vi "User_Controls.vi"() -> ()   [LabVIEW 2024]
uses:
  <vilib>/MakerHub/LINX/Public/Peripherals/Analog/Analog Read 1 Chan.vi
  <vilib>/MakerHub/LINX/Public/Peripherals/Digital/Digital Write 1 Chan.vi
  <vilib>/MakerHub/LINX/Public/Peripherals/Digital/Digital Read 1 Chan.vi
  <vilib>/MakerHub/LINX/Public/Peripherals/PWM/PWM Set Duty Cycle 1 Chan.vi
  <vilib>/MakerHub/LINX/Public/Peripherals/Digital/Digital Write N Chans.vi
  <vilib>/MakerHub/LINX/Public/Peripherals/Analog/Analog Read N Chans.vi
  <vilib>/MakerHub/LINX/Public/Peripherals/Digital/Digital Read N Chans.vi
  <vilib>/MakerHub/LINX/Private/Local IO/LinxDigitalWrite.vi
  <vilib>/MakerHub/LINX/Public/Utilities/Check Channel.vi
  <vilib>/MakerHub/LINX/Private/Local IO/LinxAnalogRead.vi
  <vilib>/MakerHub/LINX/Private/Local IO/LinxDigitalRead.vi
  <vilib>/MakerHub/LINX/Public/Utilities/Open Serial.vi
  <vilib>/MakerHub/LINX/Private/Utilties/Generate Error.vi
  <vilib>/MakerHub/LINX/Public/Peripherals/PWM/PWM Set Duty Cycle N Chans.vi
  <vilib>/MakerHub/LINX/LMH-LINX.lvlib
panel:
  in  "Tab Control":enum32{"Page 1", "Page 2"}(tab)
  in  "Log In Button":bool
  in  "Type of User :":string(combo)
  in  "Password :":string caption="Password"
  out "Led Log In":bool
  in  "Selector":bool caption="Current Mode:"
  in  "Manual Selector":bool
  out "Lower Value":bool
  in  "ON":bool
  in  "Stop Button 2":bool
  out "Curtain Position":u8(slide) scale=0.0..10.0 scale format="%.0p"
  out "Curtain Height :":dbl
  out "No. of Cycles :":u8
  in  "Motor Speed":dbl(slide) scale=0.0..23.0 scale format="%#_3g"
  in  "Down Button":bool caption="Down"
  in  "Up Button":bool
  in  "Stop":bool
  out "Stop Button":bool
  out "Upper Value":bool
  in  "Serial Port":refnum<visa-resource-name>="N/A"
  # "Curtain Interface"
  # "Version 1.0.4"
  # "Powered By:\nMecoby Inc ®"
  # "CM"
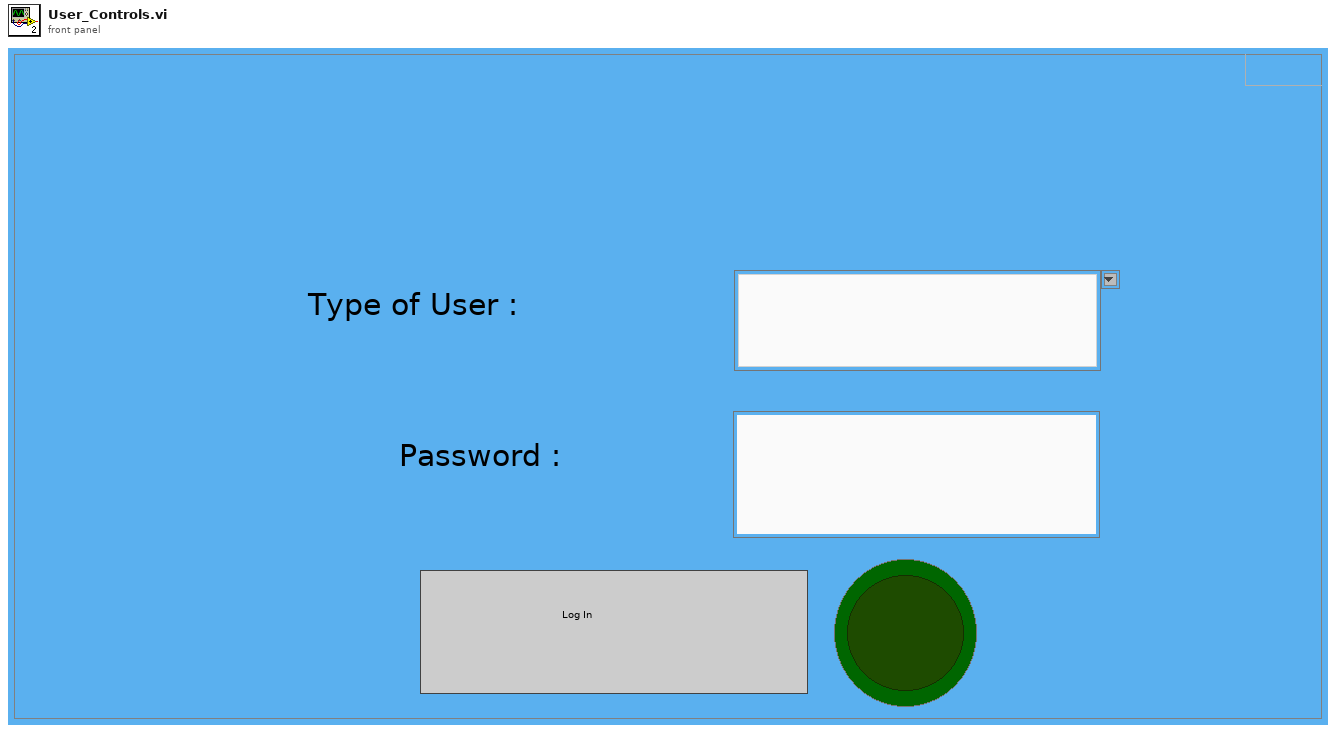
[diagram p1: front panel]
types:
  T1 = typedef "LMH-LINX.lvlib/LINX Ref.ctl" = cluster{"IO":T2, "Interface":T3, "LINX Device Config":T4}
  T2 = typedef "LMH-LINX.lvlib/Platform.ctl" = enum16{"Remote", "Local"}
  T3 = typedef "LMH-LINX.lvlib/Interface.ctl" = enum16{"Serial", "TCP"}
  T4 = typedef "LMH-LINX.lvlib/Device.lvlib/LINX Device Config.ctl" = cluster{"Interface":T3, "COM Port":refnum<visa-resource-name>, "TCP Configuration":T5, "Device Family":u8, "Device ID":u8, "Device Name":string, "TCP Ref":refnum<k5>, "Channels":T6}
  T5 = typedef "LMH-LINX.lvlib/Device.lvlib/TCP Config.ctl" = cluster{"IP Address":string, "Port":u16}
  T6 = typedef "LMH-LINX.lvlib/Channels.ctl" = cluster{"DI":u8[], "DO":u8[], "AI":u8[], "AO":u8[], "PWM":u8[], "QE":u8[], "UART":u8[], "I2C 2":u8[], "SPI":u8[], "CAN":u8[], "Servo":u8[], "AI Ref (V)":dbl, "AI Resolution (Bits)":u8, "AO Ref (V)":dbl, "AO Resolution (Bits)":u8}
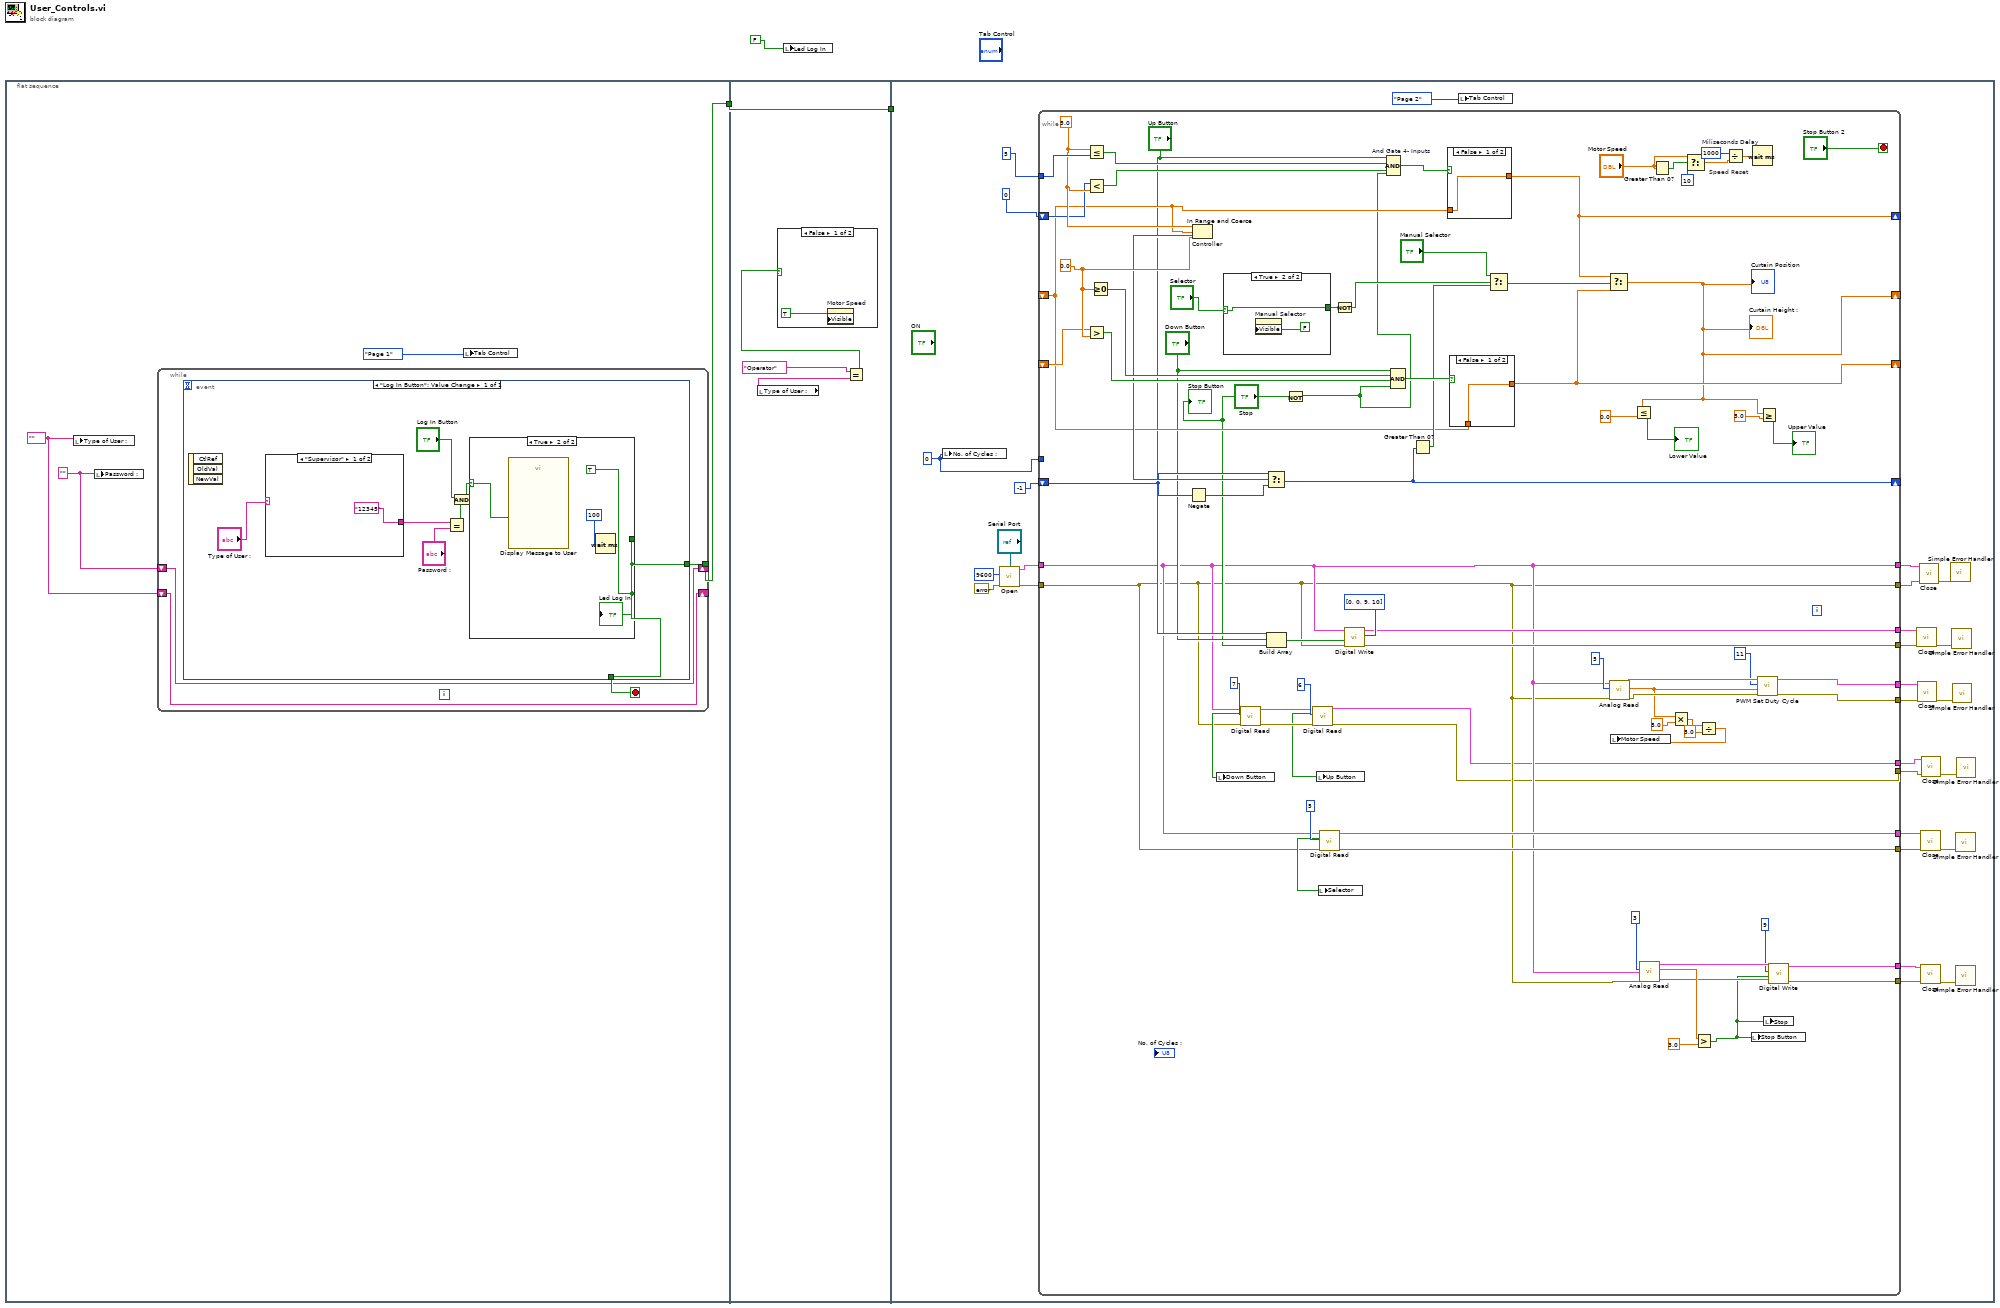
[diagram p0: block diagram]
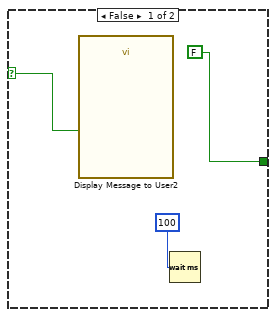
[diagram p2: hidden frame]
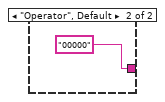
[diagram p3: hidden frame]
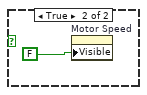
[diagram p4: hidden frame]
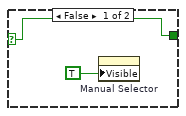
[diagram p5: hidden frame]
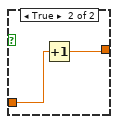
[diagram p6: hidden frame]
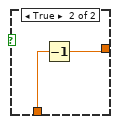
[diagram p7: hidden frame]
diagram:
  n1 = flat-sequence {
    tunnel: [w7] -> w1
    tunnel: [w27] -> w2
    tunnel: w1 -> [w27]
    tunnel: w2 -> [_]
    frame #0 {
      w5 = "" ("Type of User")
      w6 = "" ("Password")
      n2 = local write "Type of User :"(w5) -> ()
      n3 = local write "Password :"(w6) -> ()
      n4 = while {
        tunnel: [w10] -> w7
        shift-right: [w9] -> _
        shift-left: w6 -> [w9]
        shift-right: [w8] -> _
        shift-left: w5 -> [w8]
        stop <- w11 stop-if-true
        n5 = event shown="[0] \"Log In Button\": Value Change" {
          selector: _ -> [_]
          dyn-events: _ -> [_]
          timeout: _ -> [_]
          tunnel: [w12] -> w11
          tunnel: [w12] -> w10
          event "Log In Button": Value Change {
            n6 = event-data() -> ()  [unwired: 1 in, 3 out]
            n7 = case shown="\"Supervisor\"" "Type of User :" {
              tunnel: ["12345" ("x") "00000" ("x")] -> w16
              frame "Supervisor" {
              }
              frame "Operator", Default {
              }
            }
            n8 = Equal?(x=w16, y="Password :") -> (x = y?=w15:bool)
            n9 = And(x="Log In Button", y=w15) -> (x .and. y?=w14:bool)
            n10 = case shown="True" w14 {
              selector: w14 -> [w21 w24]
              tunnel: [FALSE ("OK") w22] -> w12
              frame False {
                n11 = call "Display Message to User2"("Enable"=w21) -> ()  [unwired: 9 in, 2 out]
                n12 = Wait (ms)(milliseconds to wait=u32 100) -> ()  [unwired: 1 out]
              }
              frame True {
                w22 = TRUE ("OK")
                n13 = call "Display Message to User"("Enable"=w24) -> ()  [unwired: 9 in, 2 out]
                n14 = Wait (ms)(milliseconds to wait=u32 100) -> ()  [unwired: 1 out]
                "Led Log In" <- w22
              }
            }
          }
        }
      }
      n15 = local write "Tab Control"(enum32{"Page 1", "Page 2"}."Page 1") -> ()
    }
    frame #1 {
      n16 = local read "Type of User :"() -> (w28:string)
      n17 = Equal?(x="Operator" ("Type of User"), y=w28) -> (x = y?=w30:bool)
      n18 = case shown="False" w30 {
        frame False {
          n19 = property on="Motor Speed" class="Slide (strict)"("Visible"=TRUE) -> ()  [unwired: 2 in, 2 out]
        }
        frame True {
          n20 = property on="Motor Speed" class="Slide (strict)"("Visible"=FALSE) -> ()  [unwired: 2 in, 2 out]
        }
      }
    }
    frame #2 {
      w57 = u8 0 ("No. of Cycles :")
      n21 = local write "No. of Cycles :"(w57) -> ()
      n22 = call-poly <vilib>:"Open.vi"("Error In"=errorcluster {"status"=FALSE, "code"=0, "source"=""}, "Baud Rate Override"=u32 9600, "Serial Port"="Serial Port") -> ("Error Out"=w49:errorcluster, "LINX Resource"=w51:T1)  [unwired: 6 in, 1 out]
      n23 = while {
        shift-right: [w127] -> _
        shift-left: _ -> [w114]
        shift-right: [w109] -> _
        shift-left: -1 -> [w110]
        shift-right: [w113] -> _
        shift-left: _ -> [w108]
        tunnel: u8 5 ("Curtain Position") -> [w132]
        shift-right: [w111] -> _
        shift-left: u8 0 ("Curtain Height:") -> [w112]
        tunnel: w57 -> [_]
        tunnel: [w65] -> w52
        tunnel: w51 -> [w65]
        tunnel: [w64] -> w50
        tunnel: w49 -> [w64]
        tunnel: [w96] -> w46
        tunnel: [w95] -> w45
        tunnel: [w85] -> w43
        tunnel: [w84] -> w42
        tunnel: [w62] -> w40
        tunnel: [w61] -> w39
        tunnel: [w75] -> w37
        tunnel: [w74] -> w36
        tunnel: [w67] -> w34
        tunnel: [w66] -> w33
        stop <- "Stop Button 2" stop-if-true
        w123 = 0.0 ("x")
        w124 = 5.0 ("upper limit")
        w138 = 1000  # Miliseconds Delay
        # "Speed Reset"
        n24 = Less Or Equal?(x=w124, y=w132) -> (x <= y?=w125:bool)
        n25 = Less?(x=w112, y=w124) -> (x < y?=w126:bool)
        n26 = Greater?(x=w114, y=w123) -> (0:w122:bool)
        n27 = Greater Or Equal To 0?(x=w123) -> (x >= 0?=w121:bool)
        n28 = Negate(x=w110) -> (-x=w115:i32)
        n29 = In Range and Coerce "Controller"(upper limit=w124, x=w108, lower limit=w123) -> (In Range?=w117:bool)  [unwired: 1 out]
        n30 = case shown="True" "Selector" {
          selector: "Selector" -> [w140 w142]
          tunnel: [w140 w142] -> w104
          frame False {
            n31 = property on="Manual Selector" class="Bool (strict)"("Visible"=TRUE) -> ()  [unwired: 2 in, 2 out]
          }
          frame True {
            n32 = property on="Manual Selector" class="Bool (strict)"("Visible"=FALSE) -> ()  [unwired: 2 in, 2 out]
          }
        }
        n33 = call-poly <vilib>:"Digital Read.vi"("Error In"=w64, "DI Channel"=u8 7, "LINX Resource"=w65) -> ("Error Out"=w79:errorcluster, "DI Value"=w82:bool, "LINX Resource"=w80:T1)  [unwired: 6 in]
        n34 = local write "Down Button"(w82) -> ()
        n35 = Select(t=w110, s=w117, f=w115) -> (s? t:f=w109:i32)
        n36 = Build Array("Up Button", "Down Button", "Stop") -> (w101:bool[])
        n37 = Not(x="Stop") -> (.not. x?=w107:bool)
        n38 = call-poly <vilib>:"Digital Read.vi"("Error In"=w79, "DI Channel"=u8 6, "LINX Resource"=w80) -> ("Error Out"=w61:errorcluster, "DI Value"=w78:bool, "LINX Resource"=w62:T1)  [unwired: 6 in]
        n39 = local write "Up Button"(w78) -> ()
        n40 = call-poly <vilib>:"Digital Read.vi"("Error In"=w64, "DI Channel"=u8 5, "LINX Resource"=w65) -> ("Error Out"=w74:errorcluster, "DI Value"=w76:bool, "LINX Resource"=w75:T1)  [unwired: 6 in]
        n41 = local write "Selector"(w76) -> ()
        n42 = Not(x=w104) -> (.not. x?=w118:bool)
        n43 = call-poly <vilib>:"Digital Write.vi"("Error In"=w64, "Values"=w101, "DO Channels"=u8[] [0, 0, 9, 10], "LINX Resource"=w65) -> ("Error Out"=w95:errorcluster, "LINX Resource"=w96:T1)  [unwired: 6 in]
        n44 = Compound Arithmetic op=AND "And Gate 4- Inputs"("Up Button", w125, w126, w107) -> (w130:bool)
        n45 = Compound Arithmetic op=AND("Down Button", w121, w122, w107) -> (w131:bool)
        n46 = Greater Than 0?(x=w109) -> (x > 0?=w116:bool)
        n47 = case shown="False" w130 {
          tunnel: [w143 w144] -> w111
          tunnel: w108 -> [w143 w145]
          frame False {
          }
          frame True {
            n48 = Increment(x=w145) -> (x+1=w144:dbl)
          }
        }
        n49 = case shown="False" w131 {
          tunnel: [w146 w148] -> w127
          tunnel: w108 -> [w146 w147]
          frame False {
          }
          frame True {
            n50 = Decrement(x=w147) -> (x-1=w148:dbl)
          }
        }
        n51 = Select(t="Manual Selector", s=w118, f=w116) -> (s? t:f=w119:bool)
        n52 = Select(t=w111, s=w119, f=w127) -> (s? t:f=w113:dbl)
        "Curtain Position" <- w113
        "Curtain Height :" <- w113
        n53 = call-poly <vilib>:"Analog Read.vi"("Error In"=w64, "Analog Channel"=u8 5, "LINX Resource"=w65) -> ("Error Out"=w94:errorcluster, "Voltage"=w91:dbl, "LINX Resource"=w93:T1)  [unwired: 5 in, 1 out]
        n54 = Less Or Equal?(x=w113, y=0.0) -> (x <= y?=→"Lower Value":bool)
        n55 = call-poly <vilib>:"Analog Read.vi"("Error In"=w64, "Analog Channel"=u8 3 ("DI Channel"), "LINX Resource"=w65) -> ("Error Out"=w72:errorcluster, "Voltage"=w73:dbl, "LINX Resource"=w71:T1)  [unwired: 5 in, 1 out]
        n56 = Greater Than 0?(x="Motor Speed") -> (x > 0?=w136:bool)
        n57 = Multiply(x=w91, y=5.0) -> (x*y=w90:dbl)
        n58 = Select(t="Motor Speed", s=w136, f=10) -> (s? t:f=w134:dbl)
        n59 = Greater?(x=w73, y=3.0) -> (0:w63:bool)
        n60 = Divide(x=w90, y=5.0) -> (x/y=w92:dbl)
        n61 = local write "Motor Speed"(w92) -> ()
        n62 = Divide(x=w138, y=w134) -> (x/y=w137:dbl)
        n63 = local write "Stop Button"(w63) -> ()
        n64 = Wait (ms)(milliseconds to wait=w137) -> ()  [unwired: 1 out]
        n65 = call-poly <vilib>:"PWM Set Duty Cycle.vi"("Error In"=w94, "Duty Cycle (0-1)"=w91, "PWM Channel"=u8 11, "LINX Resource"=w93) -> ("Error Out"=w84:errorcluster, "LINX Resource"=w85:T1)  [unwired: 6 in]
        n66 = Greater Or Equal?(x=w113, y=5.0) -> (x >= y?=→"Upper Value":bool)
        n67 = local write "Stop"(w63) -> ()
        n68 = call-poly <vilib>:"Digital Write.vi"("Error In"=w72, "Output Value"=w63, "DO Channel"=u8 9, "LINX Resource"=w71) -> ("Error Out"=w66:errorcluster, "LINX Resource"=w67:T1)  [unwired: 6 in]
        "Stop Button" <- "Stop"
      }
      n69 = local write "Tab Control"(enum32{"Page 1", "Page 2"}."Page 2") -> ()
      n70 = call <vilib>:"Close.vi"("Error In"=w45, "LINX Resource"=w46) -> ("Error Out"=w47:errorcluster)  [unwired: 9 in]
      n71 = call <vilib>:"Close.vi"("Error In"=w42, "LINX Resource"=w43) -> ("Error Out"=w44:errorcluster)  [unwired: 9 in]
      n72 = call <vilib>:"Close.vi"("Error In"=w50, "LINX Resource"=w52) -> ("Error Out"=w48:errorcluster)  [unwired: 9 in]
      n73 = call <vilib>:"Close.vi"("Error In"=w36, "LINX Resource"=w37) -> ("Error Out"=w38:errorcluster)  [unwired: 9 in]
      n74 = call <vilib>:"Close.vi"("Error In"=w33, "LINX Resource"=w34) -> ("Error Out"=w35:errorcluster)  [unwired: 9 in]
      n75 = call <vilib>:"Close.vi"("Error In"=w39, "LINX Resource"=w40) -> ("Error Out"=w41:errorcluster)  [unwired: 9 in]
      n76 = call <vilib>:"Simple Error Handler.vi"("error in (no error)"=w48) -> ()  [unwired: 4 in, 5 out]
      n77 = call <vilib>:"Simple Error Handler.vi"("error in (no error)"=w47) -> ()  [unwired: 4 in, 5 out]
      n78 = call <vilib>:"Simple Error Handler.vi"("error in (no error)"=w44) -> ()  [unwired: 4 in, 5 out]
      n79 = call <vilib>:"Simple Error Handler.vi"("error in (no error)"=w38) -> ()  [unwired: 4 in, 5 out]
      n80 = call <vilib>:"Simple Error Handler.vi"("error in (no error)"=w35) -> ()  [unwired: 4 in, 5 out]
      n81 = call <vilib>:"Simple Error Handler.vi"("error in (no error)"=w41) -> ()  [unwired: 4 in, 5 out]
    }
  }
  n82 = local write "Led Log In"(FALSE) -> ()
